vi "Write2CSVTest.vi"(8 "error in (no error)":errorcluster) -> (0 "error out":errorcluster)   [LabVIEW 2023, in "TestVIs.lvlib"]
uses:
  TestVIs.lvlib
  Typedefs/Cluster2DArray.ctl
  <vilib>/addons/_JKI Toolkits/Caraya/classes/Assert/Assert Equal Value_Variant.vi
  <vilib>/addons/_JKI Toolkits/Caraya/classes/Assert/Assert.lvclass
  <vilib>/addons/_JKI Toolkits/Caraya/classes/Test/Test.lvclass
  Library/Unit Testing CA1.lvlib
panel:
  # "WRITE CSV TEST"
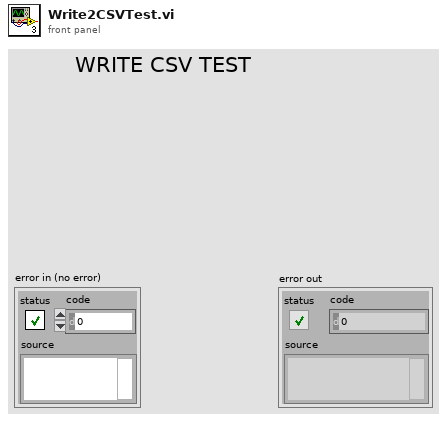
[diagram p1: front panel]
types:
  T1 = typedef "Cluster2DArray.ctl" = cluster{"Array":string[][]}
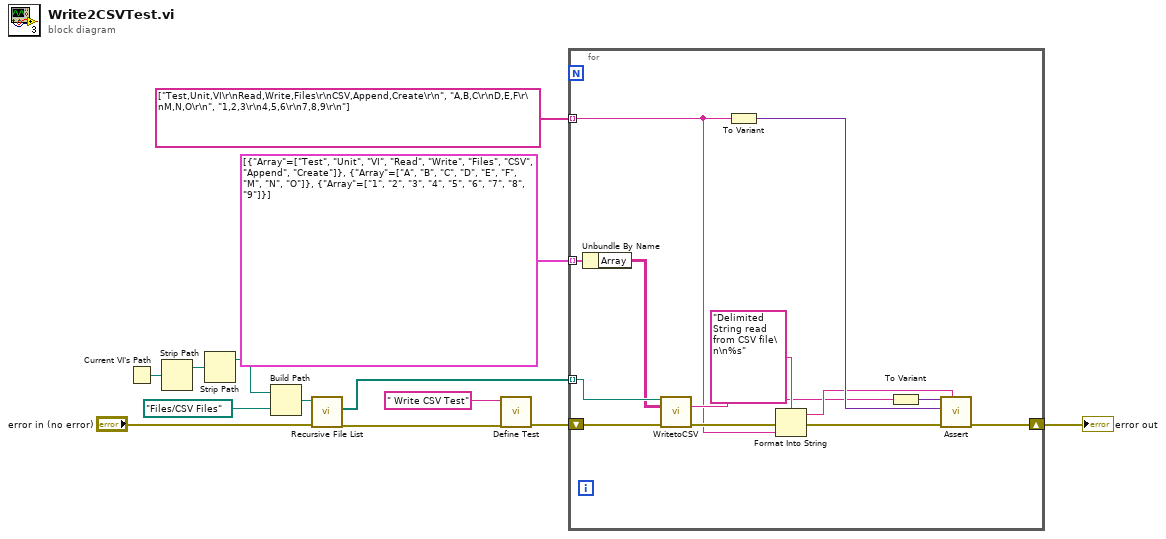
[diagram p0: block diagram]
diagram:
  n1 = Current VI's Path() -> (path=w13:path)
  n2 = Strip Path(path=w13) -> (stripped path=w10:path)  [unwired: 1 out]
  n3 = Strip Path(path=w10) -> (stripped path=w4:path)  [unwired: 1 out]
  n4 = Build Path(base path=w4, name or relative path=path "Files/CSV Files") -> (appended path=w8:path)
  n5 = call <vilib>:"Recursive File List.vi"("error in (no error)"="error in (no error)", "Folder Path"=w8) -> ("error out"=w7:errorcluster, "All Files in Dir"=w5:path[])  [unwired: 5 in, 3 out]
  n6 = call <vilib>:"Define Test.vi"("error in (no error)"=w7, "Label (VI Title)"=" Write CSV Test") -> ("error out"=w11:errorcluster)  [unwired: 8 in, 1 out]
  n7 = for {
    tunnel: w5 -> [w18] mode=indexing
    shift-right: [w21] -> w3
    shift-left: w11 -> [w20]
    tunnel: T1[] [{"Array"=[["Test", "Unit", "VI"], ["Read", "Write", "Files"], ["CSV", "Append", "Create"]]}, {"Array"=[["A", "B", "C"], ["D", "E", "F"], ["M", "N", "O"]]}, {"Array"=[["1", "2", "3"], ["4", "5", "6"], ["7", "8", "9"]]}] -> [w17] mode=indexing
    tunnel: string[] ["Test,Unit,VI\r\nRead,Write,Files\r\nCSV,Append,Create\r\n", "A,B,C\r\nD,E,F\r\nM,N,O\r\n", "1,2,3\r\n4,5,6\r\n7,8,9\r\n"] ("File/Folder Name") -> [w14] mode=indexing
    n8 = Unbundle By Name(w17) -> ("Array"=w16:string[][])
    n9 = call "WritetoCSV.vi"("File path"=w18, "Array In"=w16, "error in"=w20) -> ("spreadsheet string"=w15:string, "error out"=w19:errorcluster)  [unwired: 10 in, 1 out]
    n10 = To Variant(anything=w14) -> (Variant=w26:variant)
    n11 = Format Into String(format string="Delimited String read from CSV file\n\n%s", error in=w19, w14) -> (resulting string=w22:string, error out=w24:errorcluster)  [unwired: 1 in]
    n12 = To Variant(anything=w15) -> (Variant=w25:variant)
    n13 = call-poly <vilib>:"Assert.vi"("Label"=w22, "error in (no error)"=w24, "Y"=w26, "X"=w25) -> ("error out"=w21:errorcluster)  [unwired: 6 in, 1 out]
  }
  "error out" <- w3
